vi "HXG2DataTransFGV.vi"(7 "DataTransCtrl":T4, 8 "error in (no error)":errorcluster, 9 "Analog In":T2, 10 "Digital In":T1, 11 "Excel/Elapsed t":dbl[](array[numeric])) -> (0 "error out":errorcluster, 3 "DAQ All":T3)   [LabVIEW 2012]
uses:
  HXG2DataTrans.ctl
  Controls/HXG2_DigitalIn.ctl
  Controls/HXG2_AnalogIn.ctl
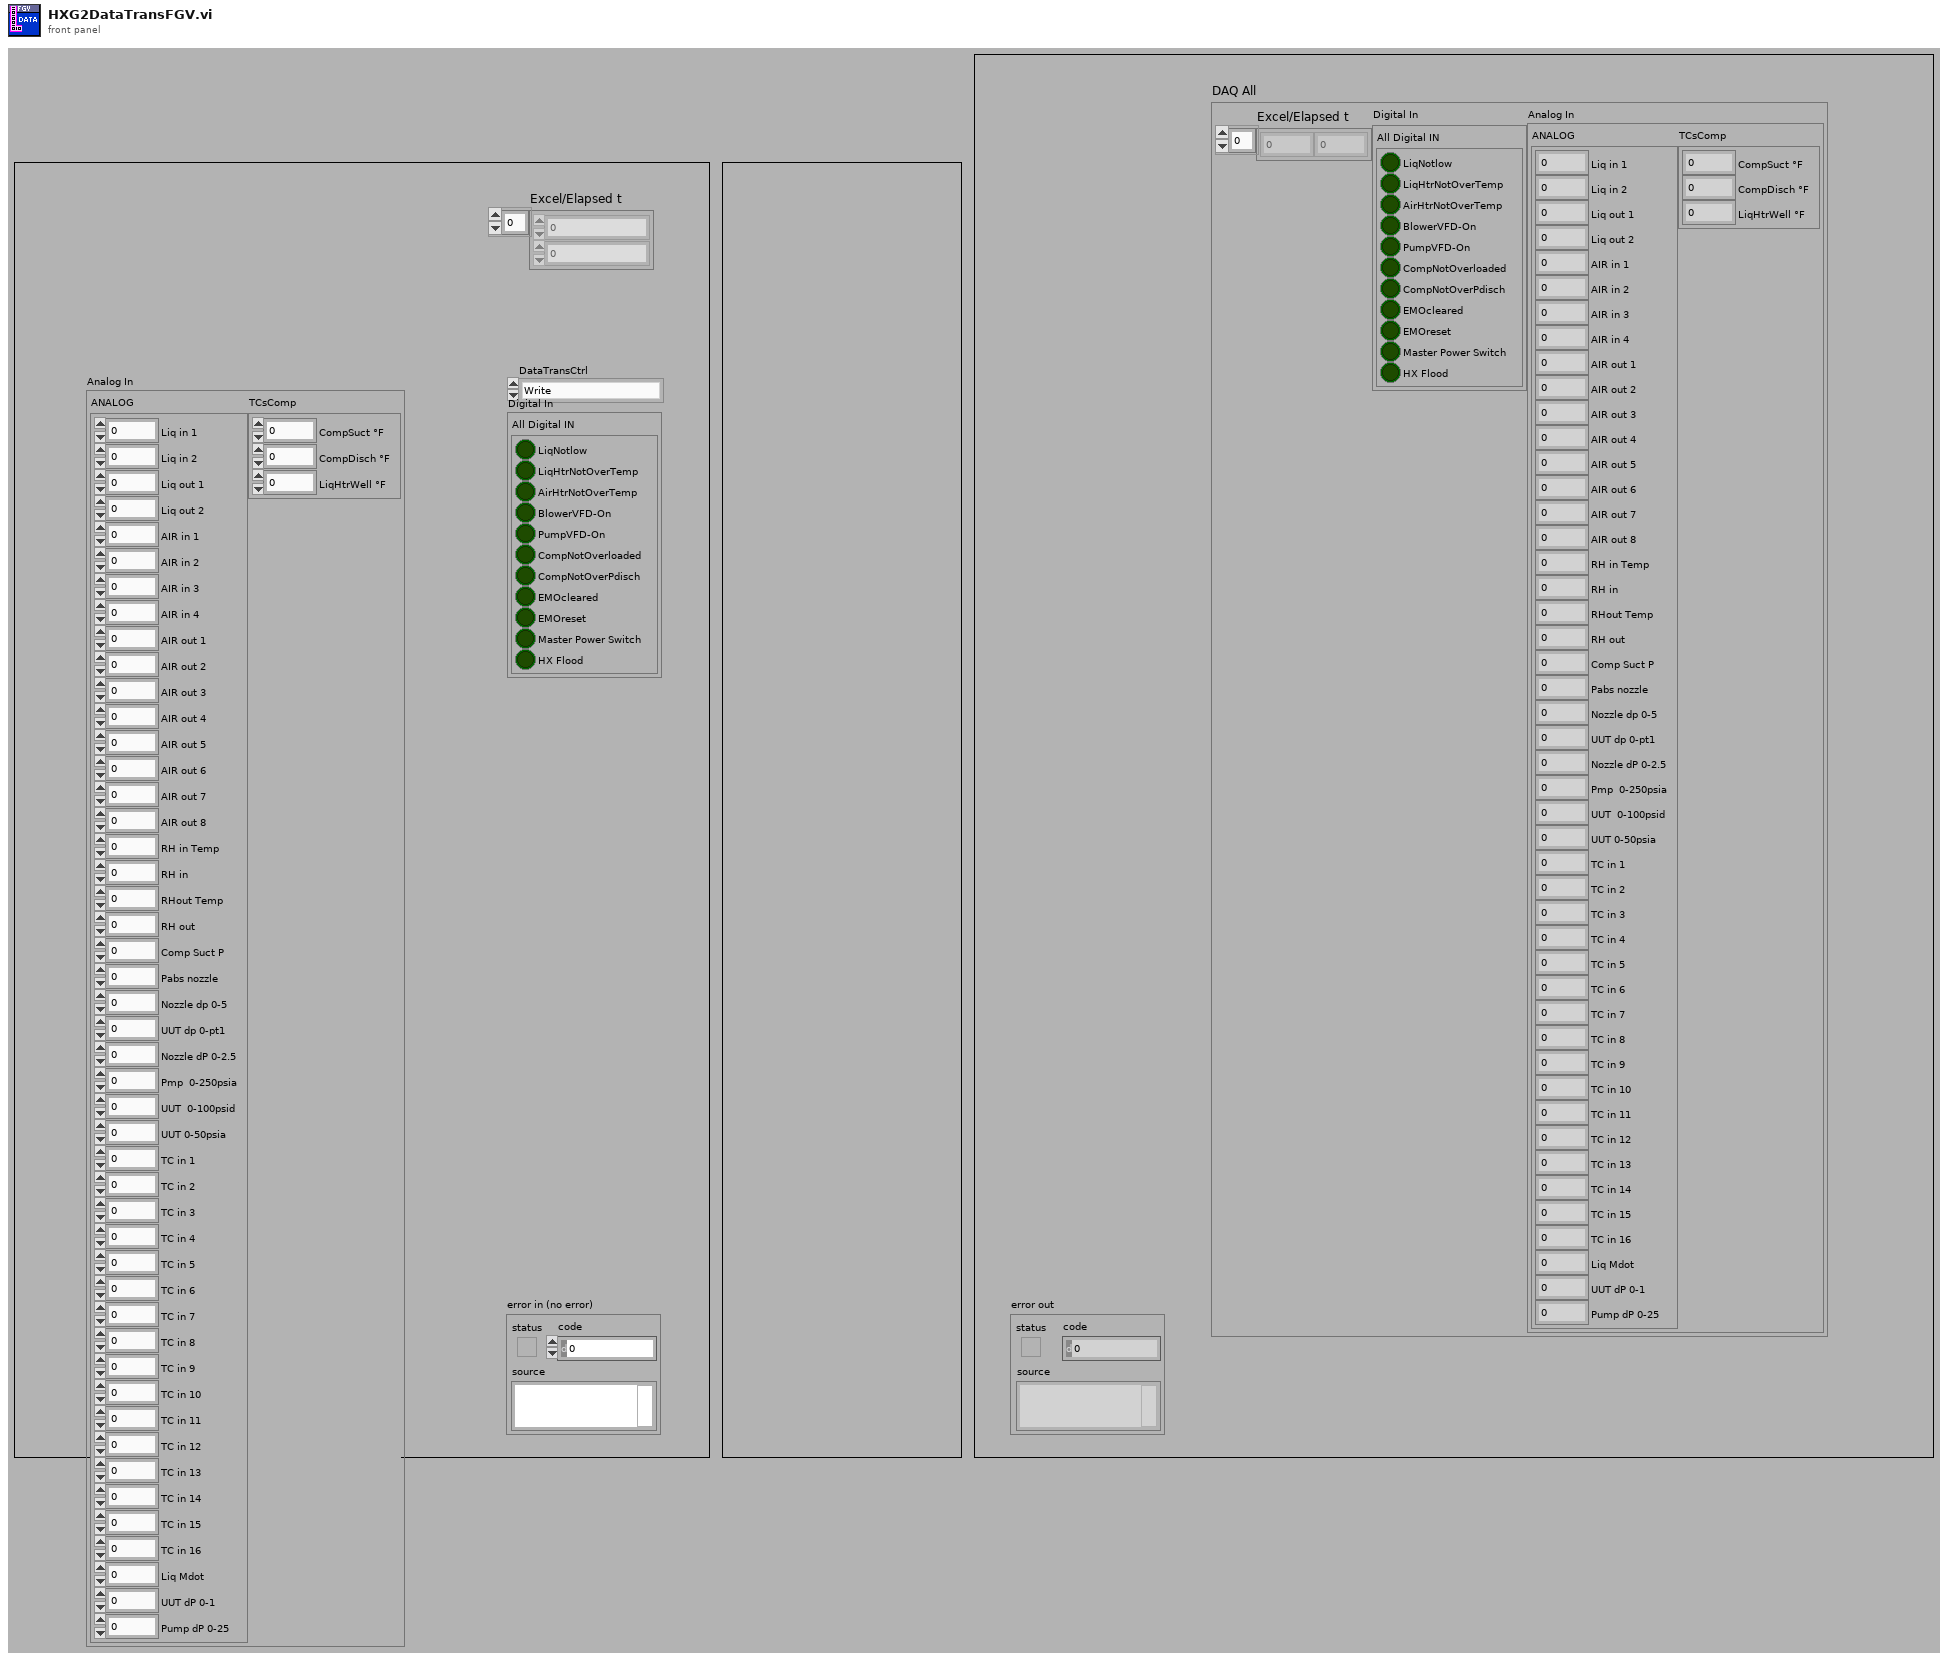
[diagram p1: front panel]
types:
  T1 = typedef "HXG2_DigitalIn.ctl" = cluster{"All Digital IN":cluster{"LiqNotlow":bool, "LiqHtrNotOverTemp":bool, "AirHtrNotOverTemp":bool, "BlowerVFD-On":bool, "PumpVFD-On":bool, "CompNotOverloaded":bool, "CompNotOverPdisch":bool, "EMOcleared":bool, "EMOreset":bool, "Master Power Switch":bool, "HX Flood":bool}}
  T2 = typedef "HXG2_AnalogIn.ctl" = cluster{"ANALOG":cluster{"Liq in 1":dbl, "Liq in 2":dbl, "Liq out 1":dbl, "Liq out 2":dbl, "AIR in 1":dbl, "AIR in 2":dbl, "AIR in 3":dbl, "AIR in 4":dbl, "AIR out 1":dbl, "AIR out 2":dbl, "AIR out 3":dbl, "AIR out 4":dbl, "AIR out 5":dbl, "AIR out 6":dbl, "AIR out 7":dbl, "AIR out 8":dbl, "RH in Temp":dbl, "RH in":dbl, "RHout Temp":dbl, "RH out":dbl, "Comp Suct P":dbl, "Pabs nozzle":dbl, "Nozzle dp 0-5":dbl, "UUT dp 0-pt1":dbl, "Nozzle dP 0-2.5":dbl, "Pmp  0-250psia":dbl, "UUT  0-100psid":dbl, "UUT 0-50psia":dbl, "TC in 1":dbl, "TC in 2":dbl, "TC in 3":dbl, "TC in 4":dbl, "TC in 5":dbl, "TC in 6":dbl, "TC in 7":dbl, "TC in 8":dbl, "TC in 9":dbl, "TC in 10":dbl, "TC in 11":dbl, "TC in 12":dbl, "TC in 13":dbl, "TC in 14":dbl, "TC in 15":dbl, "TC in 16":dbl, "Liq Mdot":dbl, "UUT dP 0-1":dbl, "Pump dP 0-25":dbl}, "TCsComp":cluster{"CompSuct °F  ":dbl, "CompDisch °F":dbl, "LiqHtrWell °F":dbl}}
  T3 = cluster{"Excel/Elapsed t":dbl[], "Digital In":T1, "Analog In":T2}
  T4 = typedef "HXG2DataTrans.ctl" = enum16{"Write", "Pass"}
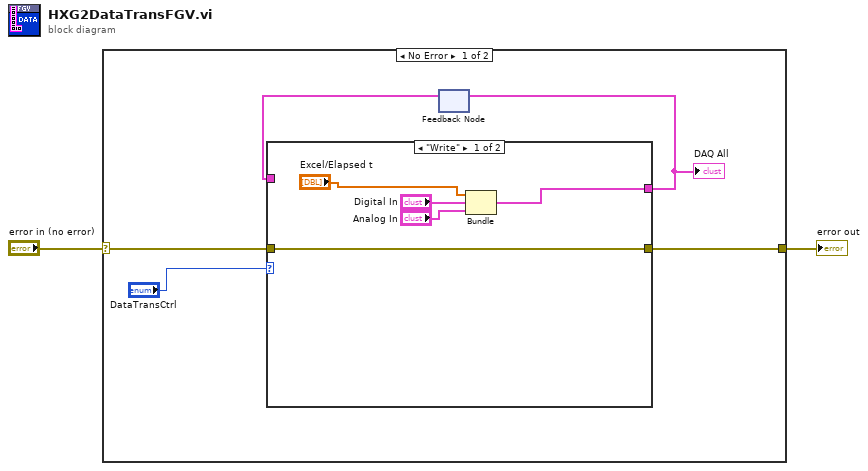
[diagram p0: block diagram]
diagram:
  n1 = case shown="No Error" "error in (no error)" {
    selector: "error in (no error)" -> [w7 w15]
    tunnel: [w6 w15] -> w1
    frame No Error {
      n2 = feedback #1() -> (w4:T3)  [unwired: 1 in]
      n3 = case shown="\"Write\"" "DataTransCtrl" {
        tunnel: w7 -> [w12 w13]
        tunnel: [w12 w13] -> w6
        tunnel: [w9 w14] -> w5
        tunnel: w4 -> [_ w14]
        frame "Write" {
          n4 = Bundle("Excel/Elapsed t"="Excel/Elapsed t", "Digital In"="Digital In", "Analog In"="Analog In") -> (w9:T3)  [unwired: 1 in]
        }
        frame "Pass" {
        }
      }
      "DAQ All" <- w5
      n5 = feedback-in #1(w5) -> ()
    }
    frame Error {
    }
  }
  "error out" <- w1
